vi "poly predictor.vi"(7 "Initialize":bool, 10 "Weight":dbl, 11 "Number of Values to Smooth":i32=600) -> (3 "Smoothed Value":dbl)   [LabVIEW 2009]
uses:
  <vilib>/Analysis/6fits.llb/Curve Fitting Criteria.ctl
  <vilib>/Analysis/NI_AALPro.lvlib
panel:
  in  "X":dbl[](array[numeric])=[1.0, 2.0, 3.0, 4.0, 5.0, 6.0, 7.0, 8.0, 9.0, 10.0, 11.0, 12.0, 13.0, 14.0, 15.0, 16.0, 17.0, 18.0, 19.0, 20.0, 21.0, 22.0, 23.0, 24.0, 25.0, 26.0, 27.0, 28.0, 29.0, 30.0, 31.0, 32.0, 33.0, 34.0, 35.0, 36.0, 37.0, 38.0, 39.0, 40.0, 41.0, 42.0, 43.0, 44.0, 45.0, 46.0, 47.0, 48.0, 49.0, 50.0, 51.0, 52.0, 53.0, 54.0, 55.0, 56.0, 57.0, 58.0, 59.0, 60.0, 61.0, 62.0, 63.0, 64.0, 65.0, 66.0, 67.0, 68.0, 69.0, 70.0, 71.0, 72.0, 73.0, 74.0, 75.0, 76.0, 77.0, 78.0, 79.0, 80.0, 81.0, 82.0, 83.0, 84.0, 85.0, 86.0, 87.0, 88.0, 89.0, 90.0, 91.0, 92.0, 93.0, 94.0, 95.0, 96.0, 97.0, 98.0, 99.0, 100.0, 101.0, 102.0, 103.0, 104.0, 105.0, 106.0, 107.0, 108.0, 109.0, 110.0, 111.0, 112.0, 113.0, 114.0, 115.0, 116.0, 117.0, 118.0, 119.0, 120.0]
  # "(assumes time is equal constant sample rate)"
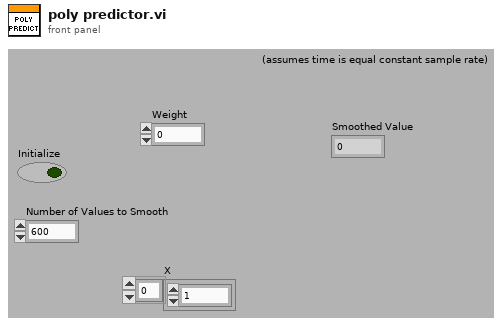
[diagram p1: front panel]
types:
  T1 = typedef "NI_AALPro.lvlib/Curve Fitting Criteria.ctl" = u16
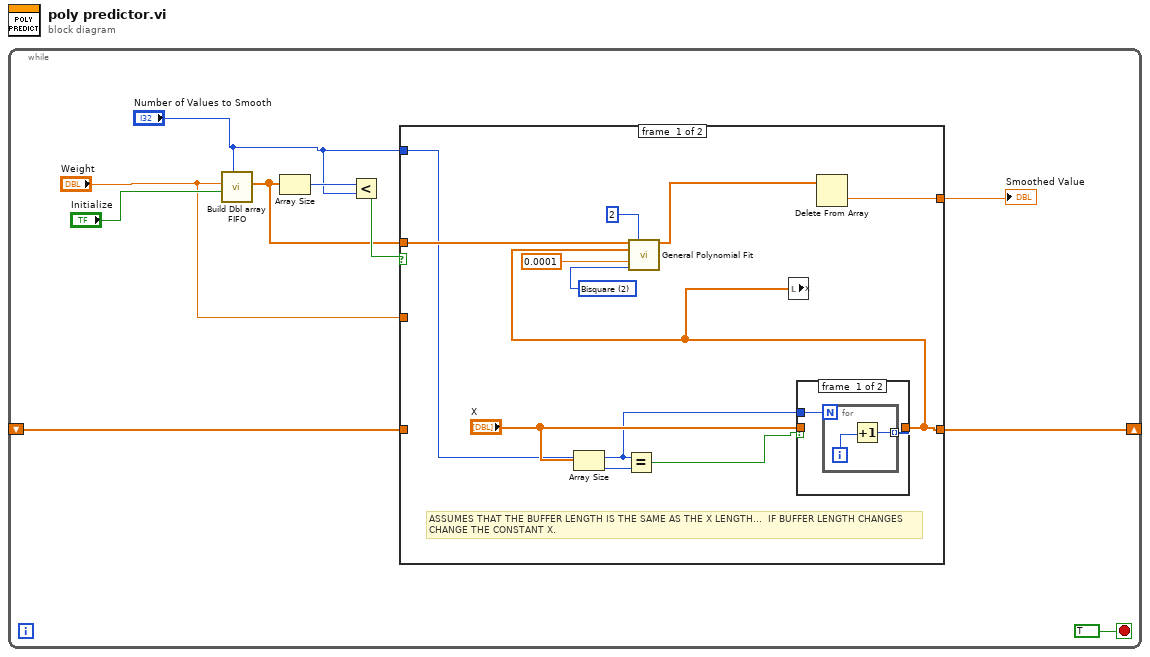
[diagram p0: block diagram]
diagram:
  n1 = while {
    shift-right: [w3] -> _
    shift-left: _ -> [w2]
    stop <- TRUE stop-if-true
    n2 = call "Build Dbl array FIFO.vi"("Max Size"="Number of Values to Smooth", "Initialize"="Initialize", "Numeric"="Weight") -> ("FIFO Array"=w7:dbl[])  [unwired: 8 in]
    n3 = Array Size(array=w7) -> (size(s)=w9:i32)
    n4 = Less?(x=w9, y="Number of Values to Smooth") -> (x < y?=w8:bool)
    n5 = case shown="False" w8 {
      tunnel: w7 -> [w18 _]
      tunnel: [w16 w28] -> w6
      tunnel: "Weight" -> [_ w28]
      tunnel: [w11 w27] -> w3
      tunnel: w2 -> [_ w27]
      tunnel: "Number of Values to Smooth" -> [w12 _]
      frame #0 {
        w20 = T1 2 items=["Least Square", "Least Absolute Residual", "Bisquare"] ("method")
        # "ASSUMES THAT THE BUFFER LENGTH IS THE SAME AS THE X LENGTH...  IF BUFFER LENGTH CHANGES\nCHANGE THE CONSTANT X."
        n6 = Array Size(array="X") -> (size(s)=w15:i32)
        n7 = Equal?(x=w12, y=w15) -> (x = y?=w14:bool)
        n8 = case shown="True" w14 {
          tunnel: [w22 w26] -> w11
          tunnel: "X" -> [_ w26]
          tunnel: w12 -> [w23 _]
          frame #0 {
            n9 = for {
              N: w23 -> [_]
              tunnel: [w24] -> w22 mode=indexing
              i -> [w25]
              n10 = Increment(x=w25) -> (x+1=w24:i32)
            }
          }
          frame #1 {
          }
        }
        n11 = call <vilib>:"General Polynomial Fit.vi"("Y"=w18, "polynomial order"=2, "X"=w11, "tolerance"=0.0001, "method"=w20) -> ("Best Polynomial Fit"=w17:dbl[])  [unwired: 7 in, 3 out]
        n12 = local write "X"(w11) -> ()
        n13 = Delete From Array(array=w17) -> (deleted portion=w16:dbl)  [unwired: 2 in, 1 out]
      }
      frame #1 {
      }
    }
    "Smoothed Value" <- w6
  }
